vi "Write ADU Packet Master.vi"(8 "error in (no error) 2":errorcluster, 9 "Modbus Data Unit":T2={"function"=1, "Data"=[]} {"function" items=["Read Discrete Inputs"=2, "Read Coils"=1, "Write Single Coil"=5, "Write Multiple Coils"=15, "Read Input Register"=4, "Read Holding Registers"=3, "Write Single Register"=6, "Write Multiple Registers"=16, "Read/Write Multiple Registers"=23, "Mask Write Register"=22, "Read FIFO Queue"=24, "Read File Record"=20, "Write File Record"=21, "Read Exception Status"=7, "Diagnostic"=8, "Get Com Event Counter"=11, "Get Com Event Log"=12, "Report Slave ID"=17, "Read Device Identification"=43]; "Data" format="%.0x"}, 10 "Unit_ID":T1={"Protocol ID"=0, "Unit ID"=1}, 11 "TCP in":refnum<class "TCP.lvclass">) -> (0 "error out 2":errorcluster, 2 "Transaction ID":u16, 3 "TCP out":refnum<class "TCP.lvclass">)   [LabVIEW 2021, in "NI_modbus_upd.lvlib"]
doc: "This uses the protocol layer to write a modbus packet to the bus, wrapped in the IP transmission data unit."
uses:
  NI_modbus_upd.lvlib
  Ctl/MB Modbus Data Unit.ctl
  Modbus Data Unit (PDU)/Function.ctl
  TCP/TCP.lvclass
  Ctl/Unit_ID.ctl
  TCP/TCP.lvclass/TCP.ctl
  <vilib>/Utility/error.llb/Clear Errors.vi
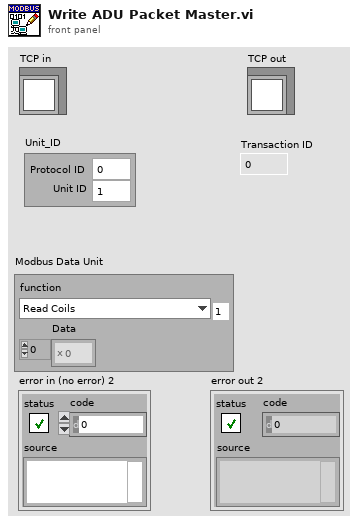
[diagram p1: front panel]
types:
  T1 = typedef "NI_modbus_upd.lvlib/Unit_ID.ctl" = cluster{"Protocol ID":u16, "Unit ID":u8}
  T2 = typedef "NI_modbus_upd.lvlib/MB Modbus Data Unit.ctl" = cluster{"function":T3, "Data":u8[]}
  T3 = typedef "NI_modbus_upd.lvlib/Function.ctl" = u8
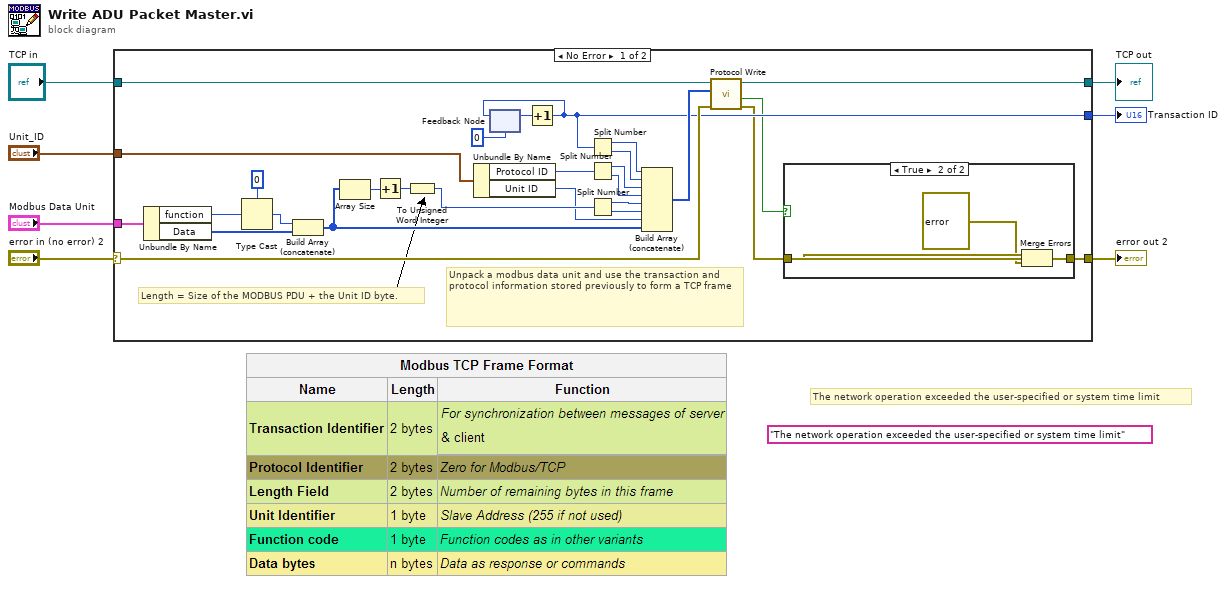
[diagram p0: block diagram]
diagram:
  (unwired) "The network operation exceeded the user-specified or system time limit"
  # "The network operation exceeded the user-specified or system time limit"
  n1 = case shown="No Error" "error in (no error) 2" {
    selector: "error in (no error) 2" -> [w17 w40]
    tunnel: "Modbus Data Unit" -> [w34 _]
    tunnel: "TCP in" -> [w19 w39]
    tunnel: [w18 w39] -> w5
    tunnel: [w8 w40] -> w3
    tunnel: [w16 _] -> w2
    tunnel: "Unit_ID" -> [w10 _]
    frame No Error {
      # "Unpack a modbus data unit and use the transaction and protocol information stored previously to form a TCP frame"
      # "Length = Size of the MODBUS PDU + the Unit ID byte."
      n2 = Unbundle By Name(w34) -> ("function"=w31:T3, "Data"=w30:u8[])
      n3 = Type Cast(type=u8 0, x=w31) -> (*(type *) &x=w33:u8)
      n4 = Build Array (concatenate)(w33, w30) -> (w21:u8[])
      n5 = Array Size(array=w21) -> (size(s)=w23:i32)
      n6 = Increment(x=w23) -> (x+1=w22:i32)
      n7 = To Unsigned Word Integer(number=w22) -> (unsigned 16bit integer=w13:u16)
      n8 = Unbundle By Name(w10) -> ("Protocol ID"=w12:u16, "Unit ID"=w11:u8)
      n9 = feedback #1(u16 0) -> (w14:u16)
      n10 = Increment(x=w14) -> (x+1=w16:u16)
      n11 = feedback-in #1(w16) -> ()
      n12 = Split Number(x=w16) -> (hi(x)=w29:u8, lo(x)=w28:u8)
      n13 = Split Number(x=w12) -> (hi(x)=w27:u8, lo(x)=w26:u8)
      n14 = Split Number(x=w13) -> (hi(x)=w25:u8, lo(x)=w24:u8)
      n15 = Build Array (concatenate)(w29, w28, w27, w26, w25, w24, w11, w21) -> (w20:u8[])
      n16 = call "Protocol Write.vi"("error in (no error)"=w17, "data"=w20, "protocol layer in"=w19) -> ("error out"=w8:errorcluster, "timed out?"=w9:bool, "protocol layer out"=w18:refnum<class "TCP.lvclass">)  [unwired: 6 in]
      n17 = case shown="True" w9 {
        tunnel: [w35 w38] -> _
        tunnel: w8 -> [w35 w37]
        frame False {
        }
        frame True {
          n18 = Merge Errors(w37, errorcluster {"status"=TRUE, "code"=56, "source"="The network operation exceeded the user-specified or system time limit"} ("error in")) -> (w38:errorcluster)
        }
      }
    }
    frame Error {
    }
  }
  "TCP out" <- w5
  "error out 2" <- w3
  "Transaction ID" <- w2
